vi "Load.vi"(10 "wait":dbl=100000.0, 11 "Stop":bool) -> ()   [LabVIEW 2019]
panel:
  out "Indicator":T1
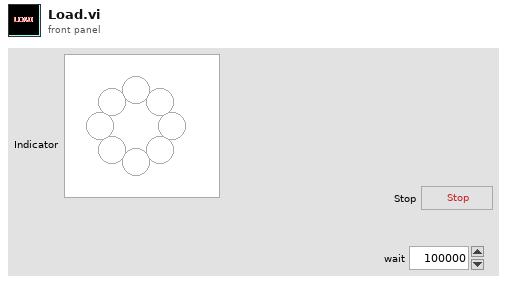
[diagram p1: front panel]
types:
  T1 = cluster{"Boolean":bool, "Boolean 2":bool, "Boolean 4":bool, "Boolean 6":bool, "Boolean 8":bool, "Boolean 7":bool, "Boolean 5":bool, "Boolean 3":bool}
  T2 = cluster{"[0]":bool, "[1]":bool, "[2]":bool, "[3]":bool, "[4]":bool, "[5]":bool, "[6]":bool, "[7]":bool}
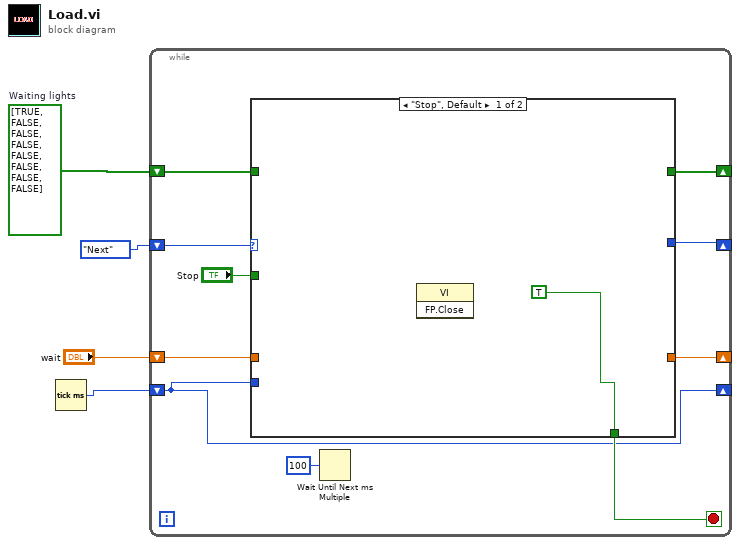
[diagram p0: block diagram]
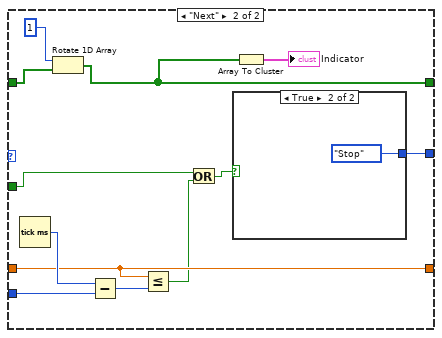
[diagram p2: hidden frame]
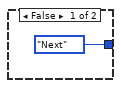
[diagram p3: hidden frame]
diagram:
  w3 = bool[] [TRUE, FALSE, FALSE, FALSE, FALSE, FALSE, FALSE, FALSE]  # Waiting lights
  n1 = Tick Count (ms)() -> (millisecond timer value=w1:u32)
  n2 = while {
    shift-right: [w10] -> _
    shift-left: enum16{"Stop", "Next"}."Next" -> [w14]
    shift-right: [w8] -> _
    shift-left: w3 -> [w13]
    shift-right: [w6] -> _
    shift-left: "wait" -> [w7]
    shift-right: [w5] -> _
    shift-left: w1 -> [w5]
    stop <- w9 stop-if-true
    n3 = case shown="\"Stop\", Default" w14 {
      tunnel: w13 -> [_ w26]
      tunnel: "Stop" -> [_ w17]
      tunnel: [_ w25] -> w10
      tunnel: [TRUE _] -> w9
      tunnel: [_ w24] -> w8
      tunnel: w7 -> [_ w19]
      tunnel: [_ w19] -> w6
      tunnel: w5 -> [_ w21]
      frame "Stop", Default {
        n4 = invoke class="VI" method="FP.Close"() -> ()  [unwired: 3 in, 3 out]
      }
      frame "Next" {
        n5 = Tick Count (ms)() -> (millisecond timer value=w22:u32)
        n6 = Rotate 1D Array(1:w26, 2:1 ("n")) -> (0:w24:bool[])
        n7 = Subtract(x=w22, y=w21) -> (x-y=w20:u32)
        n8 = Less Or Equal?(x=w19, y=w20) -> (x <= y?=w18:bool)
        n9 = Or(x=w17, y=w18) -> (x .or. y?=w16:bool)
        n10 = case shown="True" w16 {
          tunnel: [enum16{"Stop", "Next"}."Next" enum16{"Stop", "Next"}."Stop"] -> w25
          frame False {
          }
          frame True {
          }
        }
        n11 = Array To Cluster(array=w24) -> (cluster=→"Indicator":T2)
      }
    }
    n12 = Wait Until Next ms Multiple(millisecond multiple=u32 100) -> ()  [unwired: 1 out]
  }
